vi "Create NI 9474 - PWM Output.vi"(8 "error in":errorcluster, 11 "channel settings":T1[](array[typedef])) -> (0 "error out":errorcluster, 3 "NI 9474 out":refnum<class "NI 9474.lvclass">)   [LabVIEW 2020, in "Scan Engine Scripting.lvlib" / "NI 9474.lvclass"]
doc: "Creates and configures an instance of a NI-9474 counter output Pulse Width Modulation (PWM) module that can be used to set a slot in a Scan Engine custom device chassis."
uses:
  NI 9474.lvclass
  Mode Classes/Controls/pwm channel settings.ctl
  Channel Classes/PWM Output Channel/Frequency.ctl
  Mode Classes/PWM Mode/PWM Mode.lvclass
  C:/jenkins/workspace/ercat-custom-device_release_20.4/Custom Device Source/Scripting/Modules/Mode Classes/Mode/Mode.lvclass
  a71f6a1c-c12b-49d9-b8d0-ee47f7303272.vi
  Channel Classes/PWM Output Channel/PWM Output Channel.lvclass
  Scan Engine Scripting.lvlib
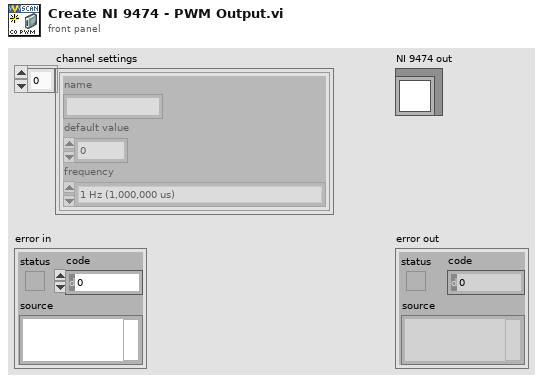
[diagram p1: front panel]
types:
  T1 = typedef "Scan Engine Scripting.lvlib/pwm channel settings.ctl" = cluster{"name":string, "default value":dbl, "frequency":T2}
  T2 = typedef "Scan Engine Scripting.lvlib/PWM Output Channel.lvclass/Frequency.ctl" = enum16{"1 Hz (1,000,000 us)", "50 Hz (20,000 us)", "250 Hz (4,000 us)", "500 Hz (2,000 us)", "1 kHz (1,000 us)", "5 kHz (200 us)", "10 kHz (100 us)", "20 kHz (50 us)"}
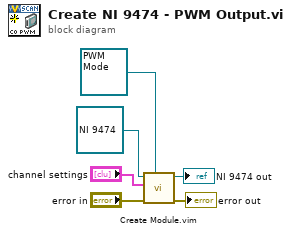
[diagram p0: block diagram]
diagram:
  n1 = call "Create Module.vim"("mode"=refnum<class "PWM Mode.lvclass"> refnum ("Scan Engine Scripting.lvlib:PWM Mode.lvclass"), "error in"="error in", "channel settings"="channel settings", "module in"=refnum<class "NI 9474.lvclass"> refnum ("Scan Engine Scripting.lvlib:NI 9474.lvclass")) -> ("error out"=→"error out":errorcluster, "module out"=→"NI 9474 out":refnum<class "NI 9474.lvclass">)  [unwired: 6 in]
